vi "Close XBox 360 Controller.vi"(8 "Rrror In":errorcluster, 11 "Device ID In":refnum<k1>) -> (0 "Error Out":errorcluster)   [LabVIEW 2011]
uses:
  _GlobalVariables&Libraries/ATV Program Global Variables.vi
  <vilib>/Utility/inputDevices.llb/closeJoystick.vi
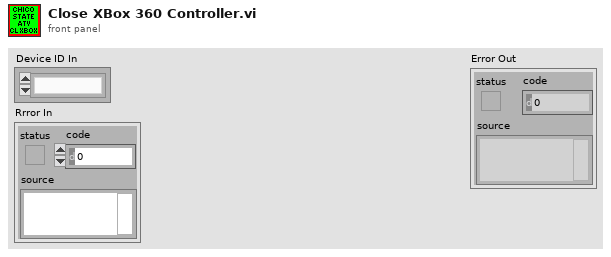
[diagram p1: front panel]
types:
  T1 = cluster{"Drive Value Output String":string, "Steer Value Output String":string, "Button A":bool, "Button B":bool, "Error Out":errorcluster, "Disable XBox Drive & Steer":bool, "Disable XBox Controller":bool, "XBOX Button Trigger Time (ms)":u32, "Button X":bool, "Button Y":bool}
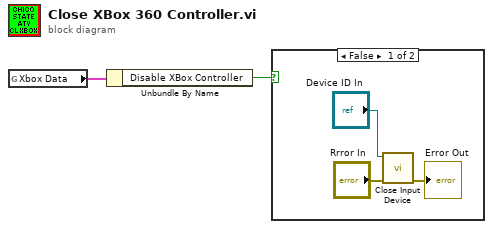
[diagram p0: block diagram]
diagram:
  n1 = global read "ATV Program Global Variables.vi" "Xbox Data"() -> (w2:T1)
  n2 = Unbundle By Name(w2) -> ("Disable XBox Controller"=w1:bool)
  n3 = case shown="False" w1 {
    frame False {
      n4 = call-poly <vilib>:"Close Input Device.vi"("error in (no error)"="Rrror In", "device ID"="Device ID In") -> ("error out"=→"Error Out":errorcluster)  [unwired: 8 in]
    }
    frame True {
    }
  }
